vi "Create-pd-actions-queue.vi"(8 "error in (no error)":errorcluster, 10 "Prefix":string) -> (0 "error out":errorcluster, 2 "ID":i32, 3 "Queue out":refnum<queue>)   [LabVIEW 2013, in "PowderDeposition.lvlib" / "PD-Main.lvclass"]
uses:
  PD-Main.lvclass
  PD-actions.ctl
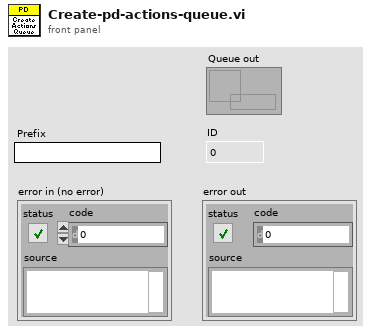
[diagram p1: front panel]
types:
  T1 = typedef "PowderDeposition.lvlib/PD-Main.lvclass/PD-actions.ctl" = enum16{"Idle", "Initialize", "Signal initialized", "Activate all motors", "Deactivate all motors", "Update motor activity", "Update selected motor", "Update motor status", "Update selected sequence", "Load sequences with dialog", "Load sequences from file", "Save sequences", "Add to sequence", "Remove from sequence", "Clear sequences", "Update available actions", "Create action", "Edit action", "Execute action", "Execute sequences", "Execute seq with assert", "Abort", "Exit"}
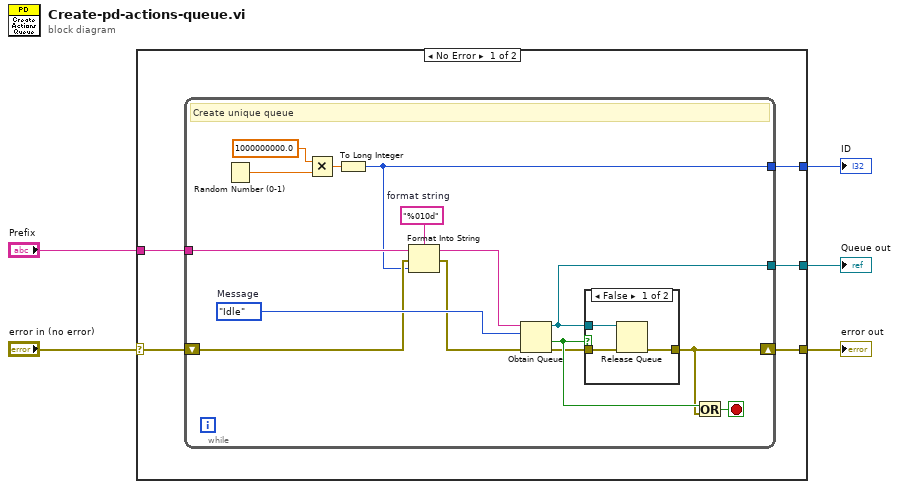
[diagram p0: block diagram]
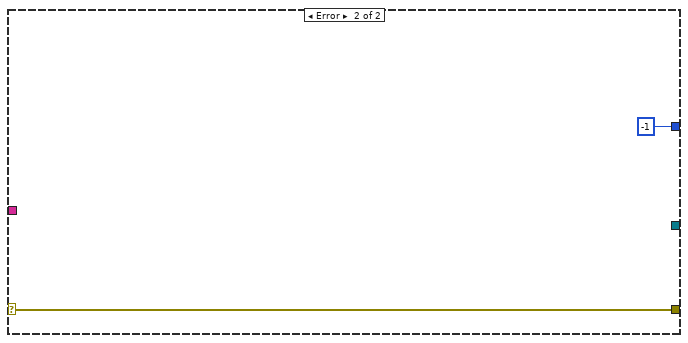
[diagram p3: hidden frame]
diagram:
  n1 = case shown="No Error" "error in (no error)" {
    selector: "error in (no error)" -> [w6 w31]
    tunnel: [w10 -1] -> w5
    tunnel: "Prefix" -> [w9 _]
    tunnel: [w8 _] -> w3
    tunnel: [w7 w31] -> w2
    frame No Error {
      n2 = while {
        shift-right: [w11] -> w7
        shift-left: w6 -> [w19]
        tunnel: [w14] -> w8
        tunnel: w9 -> [w16]
        tunnel: [w15] -> w10
        stop <- w24 stop-if-true
        w21 = "%010d"  # format string
        w25 = PD-actions."Idle"  # Message
        # "Create unique queue"
        n3 = Random Number (0-1)() -> (number: 0 to 1=w23:dbl)
        n4 = Multiply(x=1000000000.0, y=w23) -> (x*y=w20:dbl)
        n5 = To Long Integer(number=w20) -> (32bit integer=w15:i32)
        n6 = Format Into String(format string=w21, initial string=w16, error in=w19, w15) -> (resulting string=w17:string, error out=w18:errorcluster)
        n7 = Obtain Queue(name (unnamed)=w17, element data type=w25, error in (no error)=w18) -> (queue out=w14:refnum<queue>, created new?=w13:bool, error out=w12:errorcluster)  [unwired: 2 in]
        n8 = case shown="False" w13 {
          tunnel: w14 -> [w28 _]
          tunnel: w12 -> [w27 w29]
          tunnel: [w26 w29] -> w11
          frame False {
            n9 = Release Queue(queue=w28, error in (no error)=w27) -> (error out=w26:errorcluster)  [unwired: 1 in, 2 out]
          }
          frame True {
          }
        }
        n10 = Or(x=w13, y=w11) -> (x .or. y?=w24:bool)
      }
    }
    frame Error {
    }
  }
  "ID" <- w5
  "Queue out" <- w3
  "error out" <- w2
